vi "NanonisLagTest.vi"() -> ()   [LabVIEW 2019]
panel:
  in  "Z Write (m)":sgl format="%#_6p"
  out "Frame Size (m)":cluster{"Width":sgl, "Height":sgl} {"Height" format="%.2p"; "Width" format="%.2p"}
  out "Frame Origin (m)":cluster{"Xc":sgl, "Yc":sgl} {"Yc" format="%.2p"; "Xc" format="%.2p"}
  out "Current (pA)":sgl format="%#_6p"
  out "Z Read (m)":sgl format="%#_6p"
  out "Setpoint (A)":sgl format="%#_6p"
  in  "Z pen (nm)":dbl
  in  "X pen (nm)":dbl
  in  "Ring":u16(ring) items=["all", "setpoint", "zread", "current", "frame", "follow me"]
  out "elapsed time":u32
  out "tick count":u32
  in  "stop":bool
  out "Iterations":i32
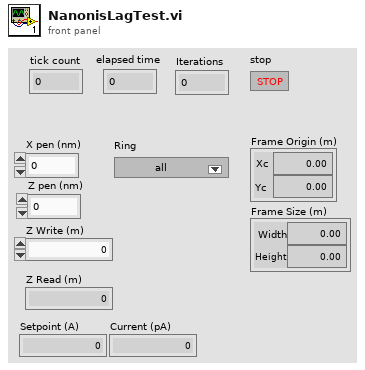
[diagram p1: front panel]
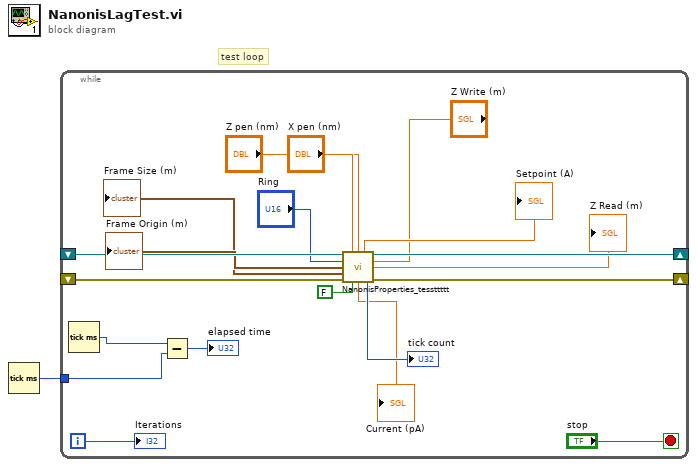
[diagram p0: block diagram]
diagram:
  # "test loop"
  n1 = Tick Count (ms)() -> (millisecond timer value=w1:u32)
  n2 = while {
    shift-right: [w19] -> _
    shift-left: _ -> [w18]
    shift-right: [w20] -> _
    shift-left: _ -> [w21]
    tunnel: w1 -> [w13]
    i -> [w17]
    stop <- "stop" stop-if-true
    n3 = Tick Count (ms)() -> (millisecond timer value=w14:u32)
    n4 = Subtract(x=w14, y=w13) -> (x-y=→"elapsed time":u32)
    n5 = call "NanonisProperties_tessttttt.vi"("Application reference"=w21, "X pen (nm)"="X pen (nm)", "Z pen (nm)"="Z pen (nm)", "Ring"="Ring", "Z Write (m)"="Z Write (m)", "Error in"=w18, "Z Write?"=FALSE) -> ("Setpoint (A)"=→"Setpoint (A)":sgl, "Application ref out"=w20:refnum<vi>, "Frame Origin (m)"=→"Frame Origin (m)":cluster{"Xc":sgl, "Yc":sgl}, "Z Read (m)"=→"Z Read (m)":sgl, "Frame Size (m)"=→"Frame Size (m)":cluster{"Width":sgl, "Height":sgl}, "Current (pA)"=→"Current (pA)":sgl, "tick count"=→"tick count":u32, "error out"=w19:errorcluster)  [unwired: 1 in]
    "Iterations" <- w17
  }
